vi "Read vi reference.vi"(9 "VI Interpreter in":refnum<class "VI Interpreter.lvclass">) -> (3 "VI Interpreter out":refnum<class "VI Interpreter.lvclass">, 4 "vi reference":refnum<vi>)   [LabVIEW 2014, in "Raspberry Pi Compatible Compiler for LabVIEW.lvlib" / "VI Interpreter.lvclass"]
uses:
  VI Interpreter.lvclass
  VI Interpreter.lvclass/VI Interpreter.ctl
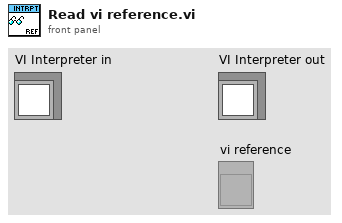
[diagram p1: front panel]
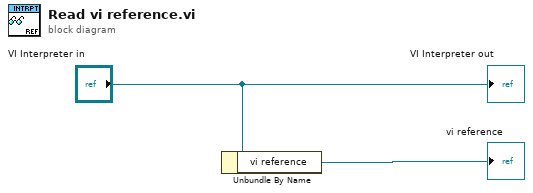
[diagram p0: block diagram]
diagram:
  n1 = Unbundle By Name("VI Interpreter in") -> ("vi reference"=→"vi reference":refnum<vi>)
  "VI Interpreter out" <- "VI Interpreter in"
